vi "Read Simulation Motor Rate.vi"(7 "motor ID":string="RightMotor,Digital Module 1,PWM 2", 9 "Invert Direction (False)":bool) -> (8 "Rate":dbl, 10 "success?":bool)   [LabVIEW 2017]
doc: "This reads the Rate scaling from the xml file. You can think of the rate as the \"gearing\" between the motor and the wheel attached to it. A smaller Rate makes the robot go faster for a given joystick input."
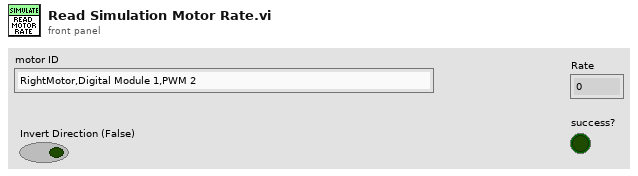
[diagram p1: front panel]
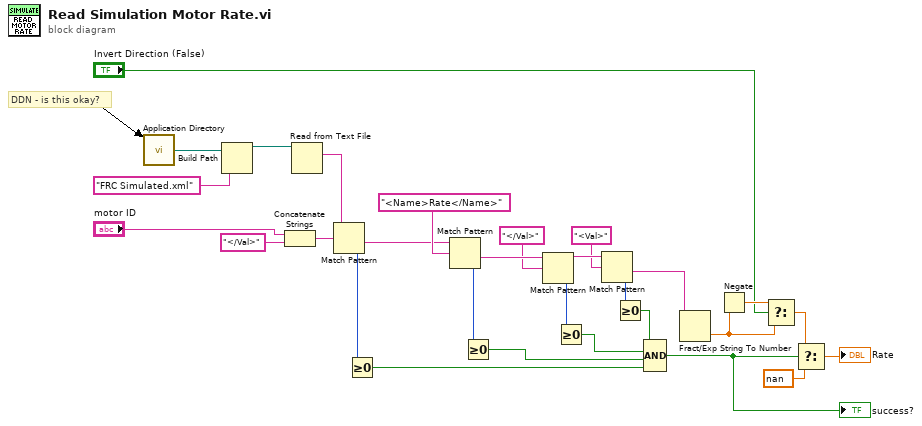
[diagram p0: block diagram]
diagram:
  # "DDN - is this okay?"
  n1 = call <vilib>:"Application Directory.vi"() -> ("Application Directory"=w21:path)
  n2 = Build Path(base path=w21, name or relative path="FRC Simulated.xml") -> (appended path=w25:path)
  n3 = Concatenate Strings("motor ID", "</Val>" ("name or relative path")) -> (w26:string)
  n4 = Read from Text File(file (use dialog)=w25) -> (text=w28:string)  [unwired: 3 in, 3 out]
  n5 = Match Pattern(string=w28, regular expression=w26) -> (after substring=w18:string, offset past match=w19:i32)  [unwired: 1 in, 2 out]
  n6 = Greater Or Equal To 0?(x=w19) -> (x >= 0?=w23:bool)
  n7 = Match Pattern(string=w18, regular expression="<Name>Rate</Name>" ("name or relative path")) -> (after substring=w15:string, offset past match=w17:i32)  [unwired: 1 in, 2 out]
  n8 = Greater Or Equal To 0?(x=w17) -> (x >= 0?=w16:bool)
  n9 = Match Pattern(string=w15, regular expression="</Val>" ("name or relative path")) -> (before substring=w13:string, offset past match=w11:i32)  [unwired: 1 in, 2 out]
  n10 = Greater Or Equal To 0?(x=w11) -> (x >= 0?=w10:bool)
  n11 = Match Pattern(string=w13, regular expression="<Val>" ("name or relative path")) -> (after substring=w9:string, offset past match=w6:i32)  [unwired: 1 in, 2 out]
  n12 = Greater Or Equal To 0?(x=w6) -> (x >= 0?=w5:bool)
  n13 = Compound Arithmetic op=AND(w5, w10, w16, w23) -> (w22:bool)
  "success?" <- w22
  n14 = Fract/Exp String To Number(string=w9) -> (number=w2:dbl)  [unwired: 3 in, 1 out]
  n15 = Negate(x=w2) -> (-x=w3:dbl)
  n16 = Select(t=w3, s="Invert Direction (False)", f=w2) -> (s? t:f=w4:dbl)
  n17 = Select(t=w4, s=w22, f=nan) -> (s? t:f=→"Rate":dbl)
